vi "Handle Error.vi"(8 "error in (no error)":errorcluster, 11 "EventRecorder in":refnum<class "EventRecorder.lvclass">) -> (0 "error out":errorcluster, 2 "stop actor?":bool=TRUE, 3 "EventRecorder out":refnum<class "EventRecorder.lvclass">)   [LabVIEW 2019, in "EventRecorder.lvlib" / "EventRecorder.lvclass"]
uses:
  EventRecorder.lvclass
  <vilib>/NI/Event Source Actor/Event Source/Event Source/Event Source.lvclass
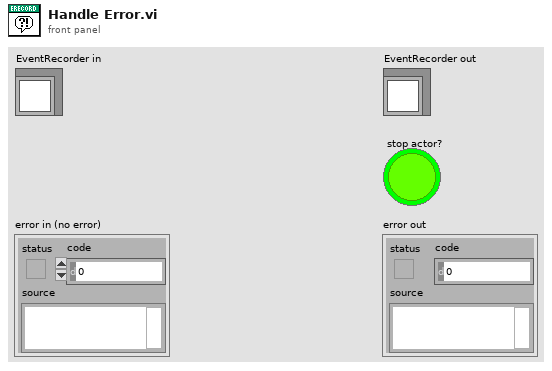
[diagram p1: front panel]
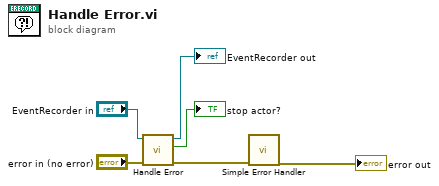
[diagram p0: block diagram]
diagram:
  n1 = call-parent "Handle Error.vi"("error in (no error)"="error in (no error)", "Actor in"="EventRecorder in") -> ("error out"=w6:errorcluster, "stop actor?"=→"stop actor?":bool, "Actor out"=→"EventRecorder out":refnum<class "EventRecorder.lvclass">)  [unwired: 7 in]
  n2 = call <vilib>:"Simple Error Handler.vi"("error in (no error)"=w6) -> ("error out"=→"error out":errorcluster)  [unwired: 4 in, 4 out]
